vi "SYSTEM.vi"() -> ()   [LabVIEW 2020]
uses:
  Control_item.ctl
panel:
  out "BuferNum1":string
  out "BuferNum2":string
  in  "OFF":bool
  out "operator":string
  out "Display":string
  in  ",":bool
  in  "=":bool
  in  "0":bool
  in  "<--":bool
  in  "C":bool
  in  "x":bool
  in  "/":bool
  in  "+":bool
  in  "-":bool
  in  "7":bool
  in  "9":bool
  in  "8":bool
  in  "5":bool
  in  "6":bool
  in  "4":bool
  in  "3":bool
  in  "2":bool
  in  "1":bool
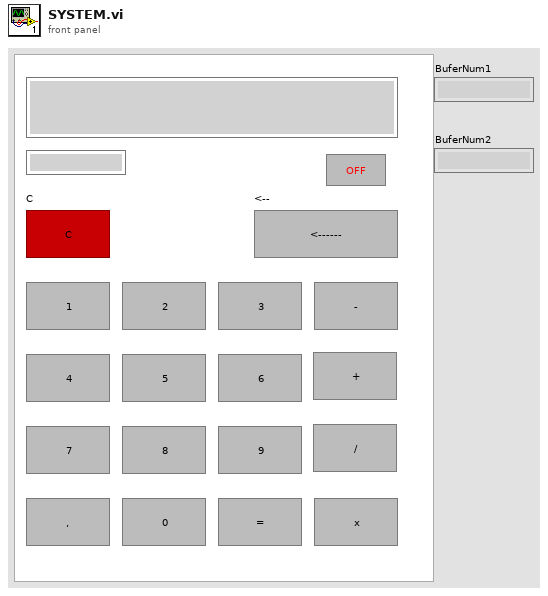
[diagram p1: front panel]
types:
  T1 = typedef "Control_item.ctl" = enum16{"Calculations", "Input Number", "Delete"}
  T2 = enum16{"Always On", "Always Off", "Off While Running"}
  T3 = cluster{"Input1":string, "Input2":string, "Operator":string}
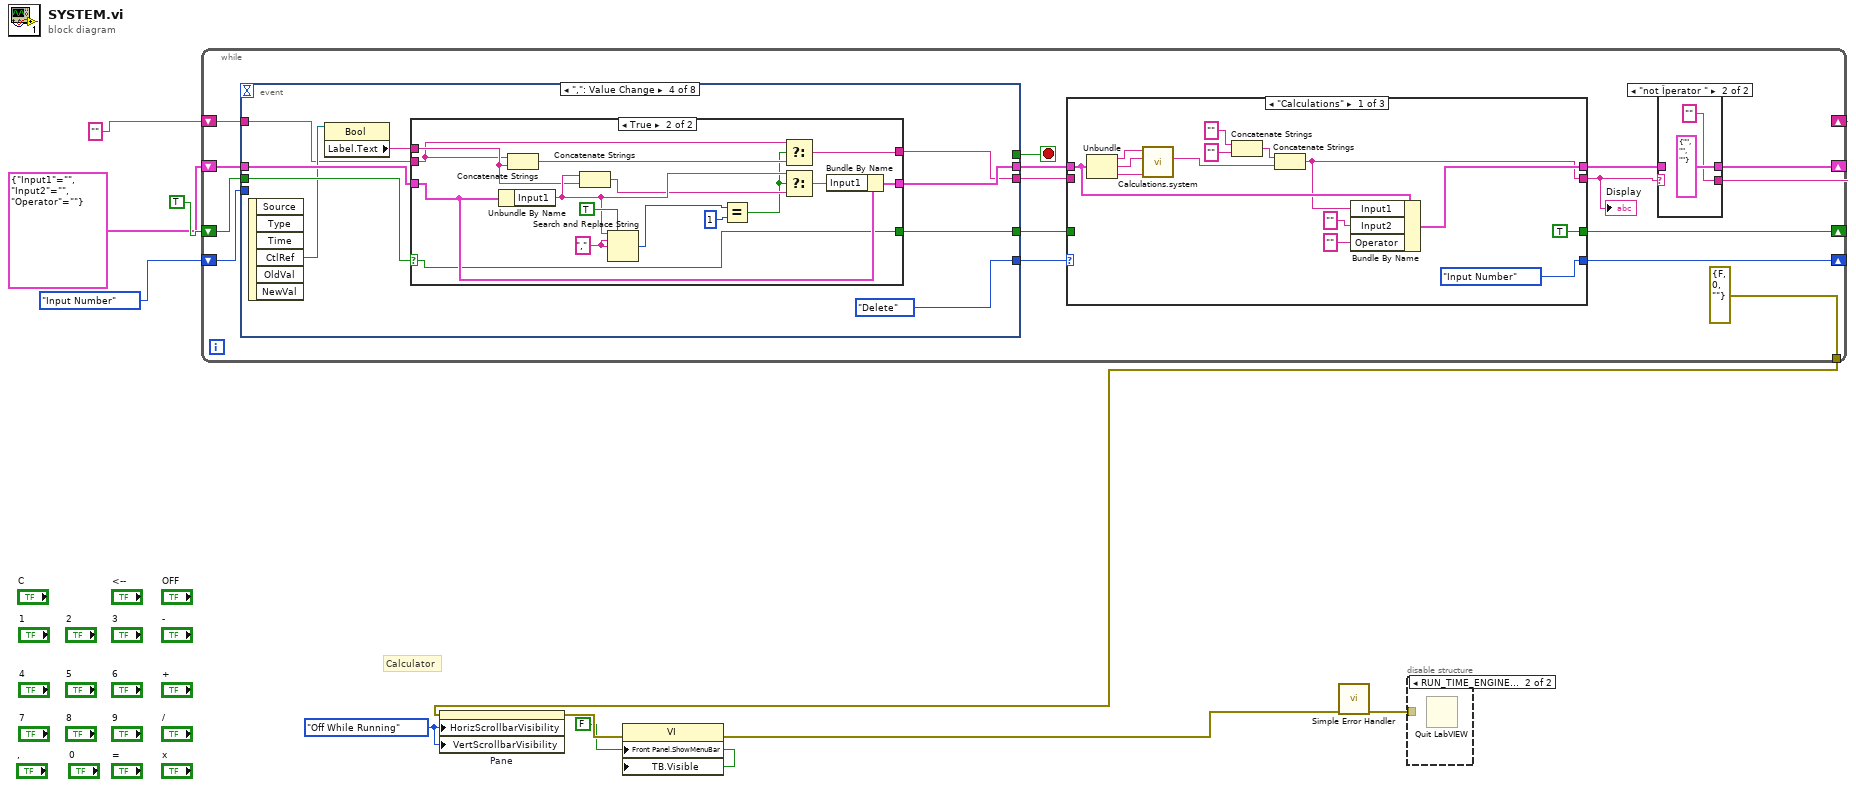
[diagram p0: block diagram]
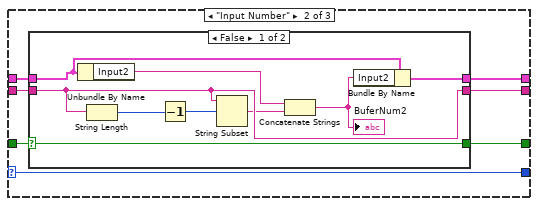
[diagram p4: hidden frame]
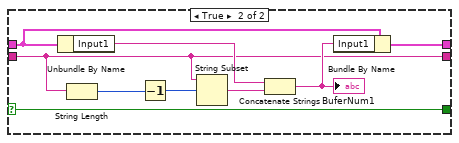
[diagram p5: hidden frame]
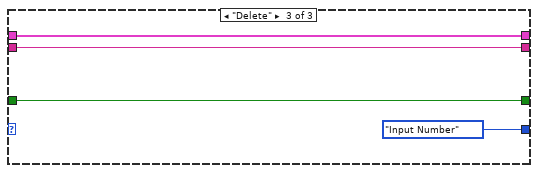
[diagram p6: hidden frame]
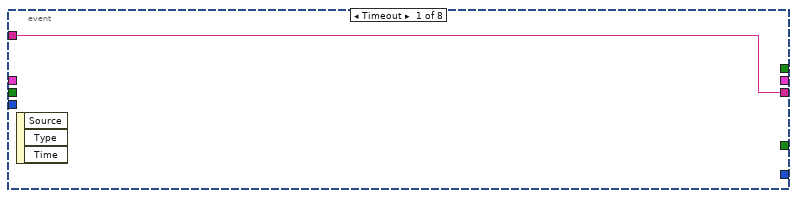
[diagram p7: hidden frame]
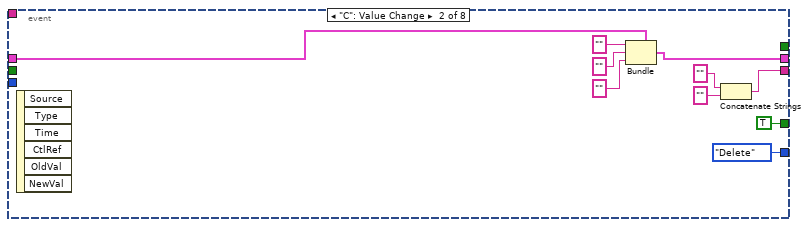
[diagram p8: hidden frame]
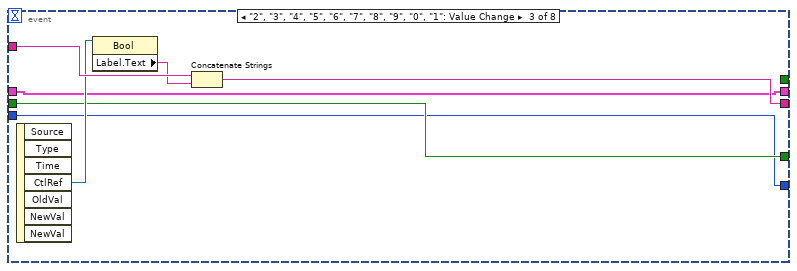
[diagram p9: hidden frame]
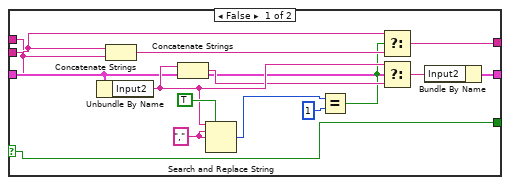
[diagram p10: hidden frame]
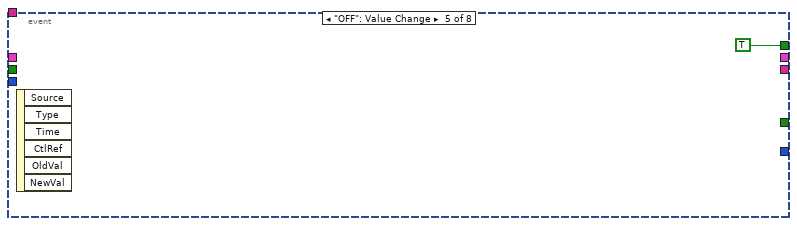
[diagram p11: hidden frame]
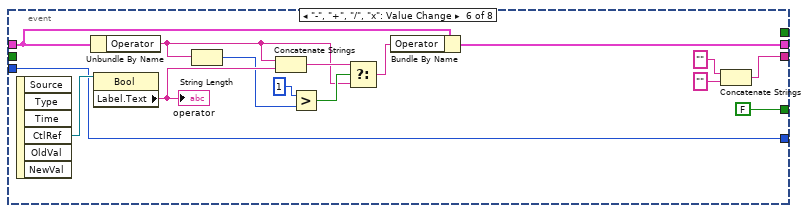
[diagram p12: hidden frame]
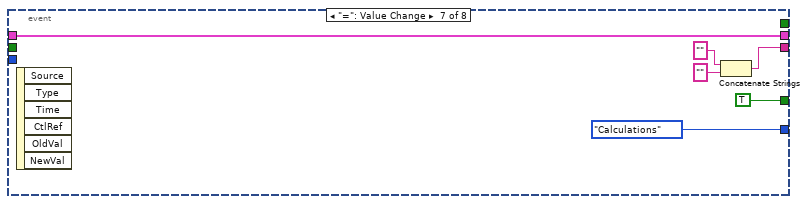
[diagram p13: hidden frame]
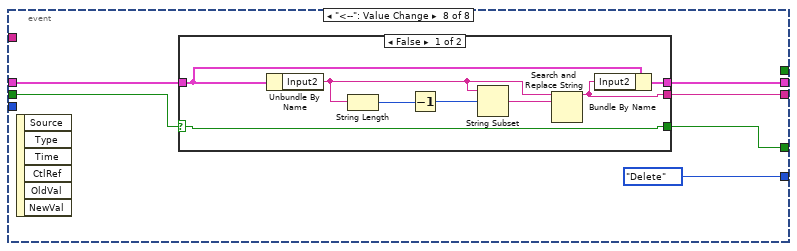
[diagram p14: hidden frame]
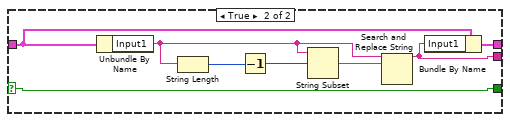
[diagram p15: hidden frame]
diagram:
  w5 = FALSE ("Front Panel Window:Show Menu Bar")
  w8 = T2."Off While Running" ("Horizontal Scrollbar Visibility")
  # "Calculator"
  n1 = while {
    shift-right: [w11] -> _
    shift-left: "" -> [w26]
    shift-right: [w16] -> _
    shift-left: TRUE -> [w25]
    shift-right: [w12] -> _
    shift-left: T3 {"Input1"="", "Input2"="", "Operator"=""} -> [w23]
    shift-right: [w15] -> _
    shift-left: Control_item."Input Number" ("States") -> [w24]
    tunnel: [errorcluster {"status"=FALSE, "code"=0, "source"=""} ("error constant")] -> w4
    stop <- w22 stop-if-true
    n2 = event shown="[3] \",\": Value Change" {
      selector: _ -> [_ _ _ _ _ _ _ _]
      dyn-events: _ -> [_ _ _ _ _ _ _ _]
      timeout: _ -> [_ _ _ _ _ _ _ _]
      tunnel: [w74 w82 w91 w94 _ w145 w152 w157] -> w19
      tunnel: w26 -> [w74 _ w90 w95 _ _ _ _]
      tunnel: w25 -> [_ _ w87 w100 _ _ _ w155]
      tunnel: [_ TRUE w87 w92 _ FALSE TRUE w156] -> w18
      tunnel: w24 -> [_ _ w86 _ _ w142 _ _]
      tunnel: [_ Control_item."Delete" ("States") w86 Control_item."Delete" ("States") _ w142 Control_item."Calculations" ("States") Control_item."Delete" ("States")] -> w17
      tunnel: w23 -> [_ w80 w85 w99 _ w141 w149 w158]
      tunnel: [_ w81 w85 w96 _ w140 w149 w153] -> w20
      tunnel: [_ _ _ _ TRUE _ _ _] -> w22
      event Timeout {
        n3 = event-data() -> ()  [unwired: 1 in, 3 out]
      }
      event "C": Value Change {
        n4 = event-data() -> ()  [unwired: 1 in, 6 out]
        n5 = Bundle(cluster=w80, "Input1"="", "Input2"="", "Operator"="") -> (w81:T3)
        n6 = Concatenate Strings("" ("string"), "" ("string")) -> (w82:string)
      }
      event "2", "3", "4", "5", "6", "7", "8", "9", "0", "1": Value Change {
        n7 = event-data() -> ("CtlRef"=w89:refnum<vi>)  [unwired: 1 in, 6 out]
        n8 = property class="Bool"(reference=w89) -> ("Label.Text"=w88:string)  [unwired: 1 in, 2 out]
        n9 = Concatenate Strings(w90, w88) -> (w91:string)
      }
      event ",": Value Change {
        n10 = event-data() -> ("CtlRef"=w98:refnum<vi>)  [unwired: 1 in, 5 out]
        n11 = property class="Bool"(reference=w98) -> ("Label.Text"=w97:string)  [unwired: 1 in, 2 out]
        n12 = case shown="True" w100 {
          selector: w100 -> [w104 w119]
          tunnel: w99 -> [w109 w124]
          tunnel: w97 -> [w107 w123]
          tunnel: [w105 w125] -> w96
          tunnel: w95 -> [w108 w121]
          tunnel: [w106 w120] -> w94
          tunnel: [w104 w119] -> w92
          frame False {
            w115 = "," ("replace string (\"\")")
            n13 = Unbundle By Name(w109) -> ("Input2"=w113:string)
            n14 = Concatenate Strings(w108, w107) -> (w110:string)
            n15 = Concatenate Strings(w113, w107) -> (w112:string)
            n16 = Search and Replace String(replace all?=TRUE ("replace all? (F)"), input string=w113, search string=w115, replace string=w115) -> (number of replacements=w102:i32)  [unwired: 4 in, 3 out]
            n17 = Equal?(x=w102, y=1) -> (x = y?=w101:bool)
            n18 = Select(t=w108, s=w101, f=w110) -> (s? t:f=w106:string)
            n19 = Select(t=w113, s=w101, f=w112) -> (s? t:f=w111:string)
            n20 = Bundle By Name(cluster=w109, "Input2"=w111) -> (w105:T3)
          }
          frame True {
            w130 = "," ("replace string (\"\")")
            n21 = Unbundle By Name(w124) -> ("Input1"=w128:string)
            n22 = Concatenate Strings(w121, w123) -> (w122:string)
            n23 = Concatenate Strings(w128, w123) -> (w127:string)
            n24 = Search and Replace String(replace all?=TRUE ("replace all? (F)"), input string=w128, search string=w130, replace string=w130) -> (number of replacements=w118:i32)  [unwired: 4 in, 3 out]
            n25 = Equal?(x=w118, y=1) -> (x = y?=w116:bool)
            n26 = Select(t=w121, s=w116, f=w122) -> (s? t:f=w120:string)
            n27 = Select(t=w128, s=w116, f=w127) -> (s? t:f=w126:string)
            n28 = Bundle By Name(cluster=w124, "Input1"=w126) -> (w125:T3)
          }
        }
      }
      event "OFF": Value Change {
        n29 = event-data() -> ()  [unwired: 1 in, 6 out]
      }
      event "-", "+", "/", "x": Value Change {
        n30 = event-data() -> ("CtlRef"=w146:refnum<vi>)  [unwired: 1 in, 5 out]
        n31 = Unbundle By Name(w141) -> ("Operator"=w133:string)
        n32 = property class="Bool"(reference=w146) -> ("Label.Text"=w139:string)  [unwired: 1 in, 2 out]
        "operator" <- w139
        n33 = String Length(string=w133) -> (length=w137:i32)
        n34 = Concatenate Strings(w133, w139) -> (w134:string)
        n35 = Greater?(x=1, y=w137) -> (0:w135:bool)
        n36 = Select(t=w134, s=w135, f=w133) -> (s? t:f=w132:string)
        n37 = Bundle By Name(cluster=w141, "Operator"=w132) -> (w140:T3)
        n38 = Concatenate Strings("" ("string"), "" ("string")) -> (w145:string)
      }
      event "=": Value Change {
        n39 = event-data() -> ()  [unwired: 1 in, 6 out]
        n40 = Concatenate Strings("" ("string"), "" ("string")) -> (w152:string)
      }
      event "<--": Value Change {
        n41 = event-data() -> ()  [unwired: 1 in, 6 out]
        n42 = case shown="False" w155 {
          selector: w155 -> [w160 w168]
          tunnel: w158 -> [w163 w171]
          tunnel: [w162 w170] -> w153
          tunnel: [w161 w169] -> w157
          tunnel: [w160 w168] -> w156
          frame False {
            n43 = Unbundle By Name(w163) -> ("Input2"=w164:string)
            n44 = String Length(string=w164) -> (length=w159:i32)
            n45 = Decrement(x=w159) -> (x-1=w166:i32)
            n46 = String Subset(string=w164, offset (0)=w166) -> (substring=w165:string)  [unwired: 1 in]
            n47 = Search and Replace String(input string=w164, search string=w165) -> (result string=w161:string)  [unwired: 6 in, 3 out]
            n48 = Bundle By Name(cluster=w163, "Input2"=w161) -> (w162:T3)
          }
          frame True {
            n49 = Unbundle By Name(w171) -> ("Input1"=w172:string)
            n50 = String Length(string=w172) -> (length=w167:i32)
            n51 = Decrement(x=w167) -> (x-1=w174:i32)
            n52 = String Subset(string=w172, offset (0)=w174) -> (substring=w173:string)  [unwired: 1 in]
            n53 = Search and Replace String(input string=w172, search string=w173) -> (result string=w169:string)  [unwired: 6 in, 3 out]
            n54 = Bundle By Name(cluster=w171, "Input1"=w169) -> (w170:T3)
          }
        }
      }
    }
    n55 = case shown="\"Calculations\"" w17 {
      selector: w17 -> [_ w45 _]
      tunnel: w20 -> [w35 w51 w71]
      tunnel: w19 -> [_ w50 w72]
      tunnel: [w34 w49 w71] -> w13
      tunnel: [w33 w48 w72] -> w14
      tunnel: w18 -> [_ w47 w70]
      tunnel: [TRUE w46 w70] -> w16
      tunnel: [Control_item."Input Number" ("States") w45 Control_item."Input Number" ("States")] -> w15
      frame "Calculations" {
        n56 = Unbundle(w35) -> ("Input1"=w42:string, "Input2"=w41:string, "Operator"=w36:string)
        n57 = call "Calculations.system.vi"("Îperator"=w36, "Number Y"=w41, "Number X"=w42) -> ("Resalt"=w39:string)  [unwired: 8 in]
        n58 = Concatenate Strings("" ("string"), "" ("string")) -> (w40:string)
        n59 = Concatenate Strings(w40, w39) -> (w33:string)
        n60 = Bundle By Name(cluster=w35, "Input1"=w33, "Input2"="", "Operator"="") -> (w34:T3)
      }
      frame "Input Number" {
        n61 = case shown="False" w47 {
          selector: w47 -> [w52 w61]
          tunnel: w50 -> [w56 w63]
          tunnel: w51 -> [w60 w64]
          tunnel: [w56 w63] -> w48
          tunnel: [w58 w62] -> w49
          tunnel: [w52 w61] -> w46
          frame False {
            n62 = Unbundle By Name(w60) -> ("Input2"=w57:string)
            n63 = String Length(string=w56) -> (length=w54:i32)
            n64 = Decrement(x=w54) -> (x-1=w53:i32)
            n65 = String Subset(string=w56, offset (0)=w53) -> (substring=w55:string)  [unwired: 1 in]
            n66 = Concatenate Strings(w57, w55) -> (w59:string)
            "BuferNum2" <- w59
            n67 = Bundle By Name(cluster=w60, "Input2"=w59) -> (w58:T3)
          }
          frame True {
            n68 = Unbundle By Name(w64) -> ("Input1"=w68:string)
            n69 = String Length(string=w63) -> (length=w66:i32)
            n70 = Decrement(x=w66) -> (x-1=w65:i32)
            n71 = String Subset(string=w63, offset (0)=w65) -> (substring=w67:string)  [unwired: 1 in]
            n72 = Concatenate Strings(w68, w67) -> (w69:string)
            "BuferNum1" <- w69
            n73 = Bundle By Name(cluster=w64, "Input1"=w69) -> (w62:T3)
          }
        }
      }
      frame "Delete" {
      }
    }
    "Display" <- w14
    n74 = case shown="\"not Îperator \"" w14 {
      selector: w14 -> [w27 _]
      tunnel: [w27 ""] -> w11
      tunnel: w13 -> [w28 _]
      tunnel: [w28 T3 {"Input1"="", "Input2"="", "Operator"=""}] -> w12
      frame "False", Default {
      }
      frame "not Îperator " {
      }
    }
  }
  n75 = property on="Pane" class="Pane"(error in=w4, "HorizScrollbarVisibility"=w8, "VertScrollbarVisibility"=w8) -> (error out=w6:errorcluster)  [unwired: 1 in, 1 out]
  n76 = property class="VI"(error in=w6, "Front Panel.ShowMenuBar"=w5, "TB.Visible"=w5) -> (error out=w3:errorcluster)  [unwired: 1 in, 1 out]
  n77 = call <vilib>:"Simple Error Handler.vi"("error in (no error)"=w3) -> ("error out"=w7:errorcluster)  [unwired: 4 in, 4 out]
  n78 = disable-structure shown="RUN_TIME_ENGINE==True" {
    disable-tunnel: w7 -> [_ _]
    frame condition #0 (active) {
    }
    frame condition #1 {
      n79 = Quit LabVIEW() -> ()  [unwired: 1 in]
    }
  }
